vi "Robotics Environment Simulator.vi"() -> ()   [LabVIEW 2012]
doc: "This VI starts and stops the environment simulator and serves as the master VI for your simulation code. Open and run this VI to display the environment simulator, or open the block diagram to view or modify simulation code."
uses:
  <vilib>/robotics/Starter Kit/2.0/Sim Host Interface/NI_Robotics_Starter Kit Host_Sim_2.0.lvclass
  <vilib>/robotics/Simulator/NI_Robotics_Simulator.lvlib
  <vilib>/robotics/Starter Kit/Host Interface/NI_Robotics_Starter Kit Host.lvclass
panel:
  out "velocidade angular((rad/s))":dbl(knob) scale=-3.0..3.0
  out "velocidade linear(m/s)":dbl(knob) scale=-4.0..4.0
  in  "?":dbl
  in  "left motor ccw velocity (rad/s)":dbl
  in  "manifest filename":string="Robotics Environment Simulator.xml"
  in  "stop":bool
  # "* Press the Run button to display the Robotics Environment Simulator.\n* Select Window>>Show Block Diagram or press <Ctrl-E> to view the block diagram, where you can add or modify simulation code. Add controls and indicators to the front panel of this VI to pass data into and out of the simulation code.\n* The manifest file must exist in same directory as the .lvproj file."
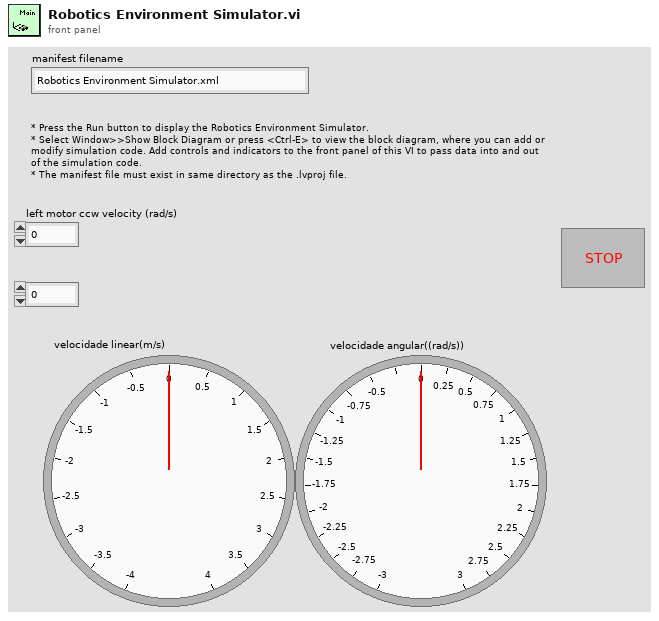
[diagram p1: front panel]
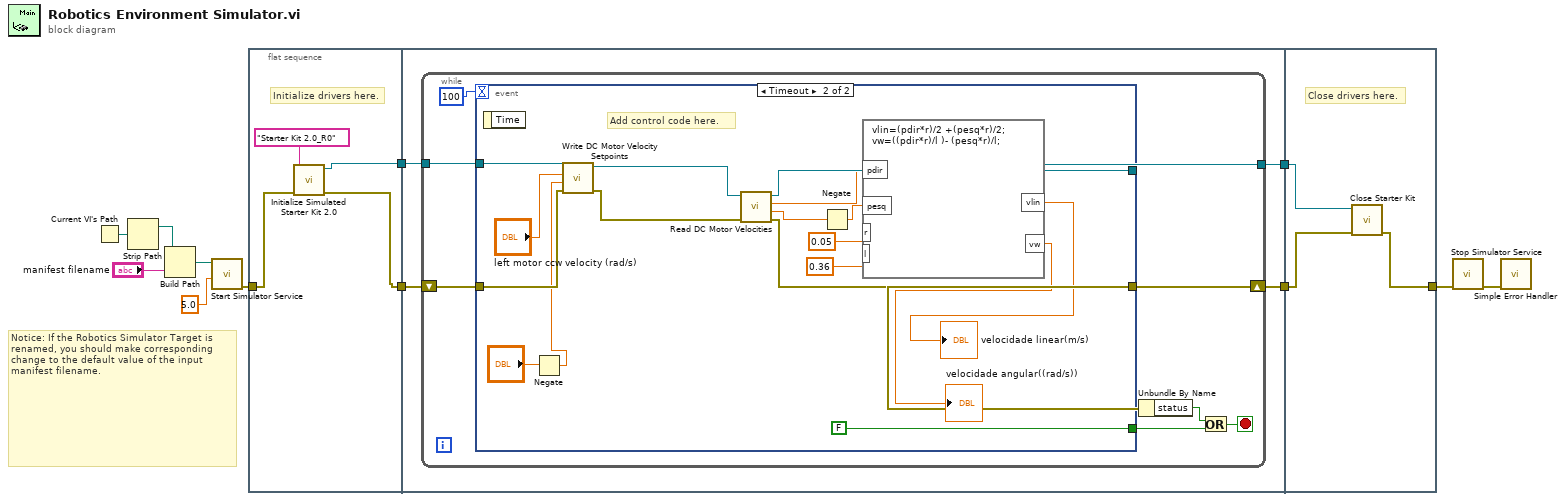
[diagram p0: block diagram]
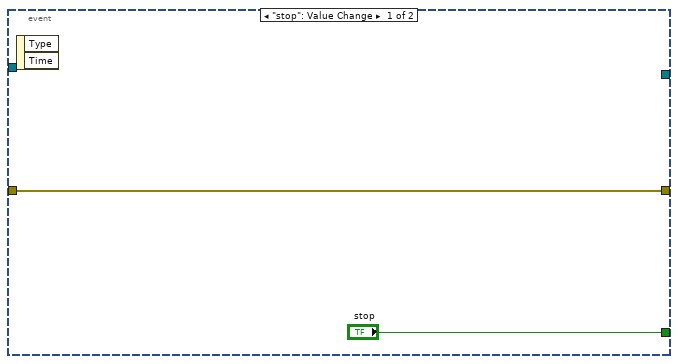
[diagram p2: hidden frame]
diagram:
  # "Notice: If the Robotics Simulator Target is renamed, you should make corresponding change to the default value of the input manifest filename."
  n1 = Current VI's Path() -> (path=w10:path)
  n2 = Strip Path(path=w10) -> (stripped path=w9:path)  [unwired: 1 out]
  n3 = Build Path(base path=w9, name or relative path="manifest filename") -> (appended path=w8:path)
  n4 = call <vilib>:"Start Simulator Service.vi"("step size (ms)"=5.0 ("stepsize(ms)"), "manifest file"=w8) -> ("error out"=w5:errorcluster)  [unwired: 9 in]
  n5 = flat-sequence {
    tunnel: w5 -> [w15]
    tunnel: [w14] -> w4
    tunnel: [w13] -> w2
    tunnel: w4 -> [w19]
    tunnel: [w20] -> w3
    tunnel: w2 -> [w18]
    tunnel: [w17] -> w1
    tunnel: [w48] -> w11
    tunnel: w3 -> [w50]
    tunnel: w1 -> [w49]
    frame #0 {
      # "Initialize drivers here."
      n6 = call <vilib>:"Initialize Simulated Starter Kit 2.0.vi"("error in (no error)"=w15, "robot ID"="Starter Kit 2.0_R0") -> ("error out"=w14:errorcluster, "simulated starter kit host 2.0 out"=w13:refnum<class "NI_Robotics_Starter Kit Host_Sim_2.0.lvclass">)  [unwired: 8 in]
    }
    frame #1 {
      n7 = while {
        shift-right: [w24] -> w20
        shift-left: w19 -> [w27]
        tunnel: w18 -> [w22]
        tunnel: [w21] -> w17
        stop <- w25 stop-if-true
        n8 = event shown="[1] Timeout" {
          selector: _ -> [_ _]
          dyn-events: _ -> [_ _]
          timeout: 100 -> [_ _]
          tunnel: ["stop" FALSE ("stop")] -> w26
          tunnel: [w29 w37] -> w24
          tunnel: w27 -> [w29 w44]
          tunnel: w22 -> [_ w46]
          tunnel: [_ w40] -> w21
          event "stop": Value Change {
            n9 = event-data() -> ()  [unwired: 1 in, 2 out]
          }
          event Timeout {
            # "Add control code here."
            n10 = event-data() -> ()  [unwired: 1 in, 1 out]
            n11 = Negate(x="?") -> (-x=w42:dbl)
            n12 = call <vilib>:"Write DC Motor Velocity Setpoints.vi"("error in (no error)"=w44, "right motor ccw velocity (rad/s)"=w42, "left motor ccw velocity (rad/s)"="left motor ccw velocity (rad/s)", "starter kit host in"=w46) -> ("error out"=w38:errorcluster, "starter kit host out"=w41:refnum<class "NI_Robotics_Starter Kit Host_Sim_2.0.lvclass">)  [unwired: 6 in]
            n13 = call <vilib>:"Read DC Motor Velocities.vi"("error in (no error)"=w38, "starter kit host in"=w41) -> ("error out"=w37:errorcluster, "right motor ccw velocity (rad/s)"=w39:dbl, "left motor ccw velocity (rad/s)"=w36:dbl, "starter kit host out"=w40:refnum<class "NI_Robotics_Starter Kit Host_Sim_2.0.lvclass">)  [unwired: 6 in]
            n14 = Negate(x=w39) -> (-x=w33:dbl)
            n15 = formula code="vlin=(pdir*r)/2 +(pesq*r)/2;\nvw=((pdir*r)/l )- (pesq*r)/l;"("pdir"=w36, "pesq"=w33, "r"=0.05 ("input variable"), "l"=0.36 ("input variable")) -> ("vlin"=→"velocidade linear(m/s)":dbl, "vw"=→"velocidade angular((rad/s))":dbl)
          }
        }
        n16 = Unbundle By Name(w24) -> ("status"=w23:bool)
        n17 = Or(x=w23, y=w26) -> (x .or. y?=w25:bool)
      }
    }
    frame #2 {
      # "Close drivers here."
      n18 = call-dynamic "Close Starter Kit.vi"("error in (no error)"=w50, "starter kit host in"=w49) -> ("error out"=w48:errorcluster)  [unwired: 9 in]
    }
  }
  n19 = call <vilib>:"Stop Simulator Service.vi"("error in (no error)"=w11) -> ("error out"=w6:errorcluster)  [unwired: 10 in]
  n20 = call <vilib>:"Simple Error Handler.vi"("error in (no error)"=w6) -> ()  [unwired: 4 in, 5 out]
